vi "Run.vi"(0 "Status输入":T1, 5 "错误输入（无错误）":errorcluster) -> (14 "Status输出":T1, 15 "Lamp":bool[](array[boolean]), 19 "错误输出":errorcluster)   [LabVIEW 2013]
uses:
  Status.ctl
  Step.ctl
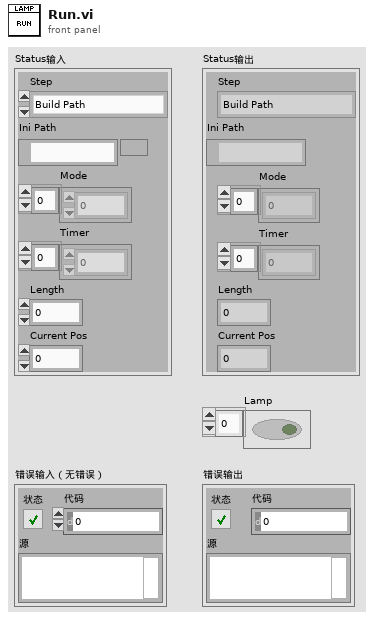
[diagram p1: front panel]
types:
  T1 = typedef "Status.ctl" = cluster{"Step":T2, "Ini Path":path, "Mode":u32[], "Timer":dbl[], "Length":i32, "Current Pos":i32}
  T2 = typedef "Step.ctl" = enum16{"Build Path", "Read Ini", "Run"}
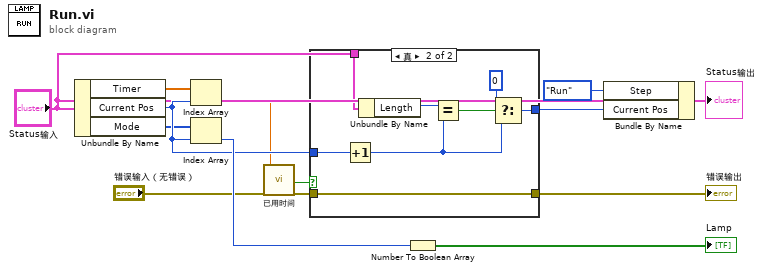
[diagram p0: block diagram]
diagram:
  n1 = Unbundle By Name("Status输入") -> ("Timer"=w8:dbl[], "Current Pos"=w12:i32, "Mode"=w11:u32[])
  n2 = Index Array(array=w8, index=w12) -> (element=w9:dbl)
  n3 = Index Array(array=w11, index=w12) -> (element=w13:u32)
  n4 = call "已用时间"("Time Target (s)"=w9, "error in (no error)"="错误输入（无错误）") -> ("Time has Elapsed"=w1:bool, "error out"=w4:errorcluster)  [unwired: 10 in, 6 out]
  n5 = case shown="真" w1 {
    tunnel: [w15 w21] -> w14
    tunnel: [w16 w20] -> w5
    tunnel: w4 -> [w16 w20]
    tunnel: w12 -> [w15 w19]
    tunnel: "Status输入" -> [_ w18]
    frame False {
    }
    frame True {
      n6 = Increment(x=w19) -> (x+1=w22:i32)
      n7 = Unbundle By Name(w18) -> ("Length"=w17:i32)
      n8 = Equal?(x=w17, y=w22) -> (x = y?=w24:bool)
      n9 = Select(t=0, s=w24, f=w22) -> (s? t:f=w21:i32)
    }
  }
  "错误输出" <- w5
  n10 = Number To Boolean Array(number=w13) -> (Boolean array=→"Lamp":bool[])
  n11 = Bundle By Name(cluster="Status输入", "Step"=Step."Run", "Current Pos"=w14) -> (→"Status输出":T1)
